vi "log analysis_gps.vi"() -> ()   [LabVIEW 2019] (continued)
INS_RTKFIXED,37.37077766145,126.72401317567,9.8633,22.3000,-0.2009,0.2209,0.0247,-0.192396038,1.572189477,119.250218807,0.6084,0.3900,0.7185,0.1389,0.1090,0.0824,0.1462,0.1512,5.0046,0f000001,0*0ea2a365\n\t", "INSPVAXA,USB3,0,52.5,FINESTEERING,2107,282225.550,02000000,471d,15824;INS_ALIGNMENT_COMPLETE,INS_RTKFIXED,37.37077734941,126.72401466448,9.8621,22.3000,-0.1997,0.2260,0.0207,-0.108448502,1.711031011,118.230862766,0.6084,0.3900,0.7185,0.1389,0.1090,0.0824,0.1462,0.1512,5.0046,0f000001,0*0e52b076\n\t", "INSPVAXA,USB3,0,48.5,FINESTEERING,2107,282226.050,02000000,471d,15824;INS_ALIGNMENT_COMPLETE,INS_RTKFIXED,37.37077704777,126.72401614595,9.8618,22.3000,-0.1720,0.2084,0.0247,-0.161231391,1.488834735,117.043709795,0.5373,0.3399,0.6690,0.1307,0.1036,0.0789,0.1454,0.1502,5.0054,0f000001,0*01dce4f3\n\t", "INSPVAXA,USB3,0,48.5,FINESTEERING,2107,282227.050,02000000,471d,15824;INS_ALIGNMENT_COMPLETE,INS_RTKFIXED,37.37077593278,126.72401891596,9.8631,22.3000,-0.1697,0.2262,0.0181,-0.178975170,1.493639019,115.812677176,0.5005,0.3171,0.6343,0.1279,0.1027,0.0771,0.1451,0.1499,5.0056,0f000001,0*b5f48b56\n\t", "INSPVAXA,USB3,0,51.0,FINESTEERING,2107,282227.550,02000000,471d,15824;INS_ALIGNMENT_COMPLETE,INS_RTKFIXED,37.37077534199,126.72402027291,9.8655,22.3000,-0.1792,0.2154,0.0259,-0.205196219,1.587681370,115.700553222,0.5005,0.3171,0.6343,0.1279,0.1027,0.0771,0.1451,0.1499,5.0056,0f000001,0*9a4eb5a2\n\t", "INSPVAXA,USB3,0,51.0,FINESTEERING,2107,282228.050,02000000,471d,15824;INS_ALIGNMENT_COMPLETE,INS_RTKFIXED,37.37077473925,126.72402159293,9.8669,22.3000,-0.1676,0.2065,0.0190,-0.168899804,1.509556154,115.821588566,0.4803,0.3065,0.6087,0.1271,0.1026,0.0763,0.1447,0.1496,5.0053,0f000001,0*25784804\n\t", "INSPVAXA,USB3,0,52.5,FINESTEERING,2107,282228.550,02000000,471d,15824;INS_ALIGNMENT_COMPLETE,INS_RTKFIXED,37.37077412906,126.72402288572,9.8668,22.3000,-0.1602,0.2130,0.0258,-0.196596636,1.388177172,115.979386072,0.4803,0.3065,0.6087,0.1271,0.1026,0.0763,0.1447,0.1496,5.0053,0f000001,0*cbeb8b2e\n\t", "INSPVAXA,USB3,0,50.5,FINESTEERING,2107,282229.050,02000000,471d,15824;INS_ALIGNMENT_COMPLETE,INS_RTKFIXED,37.37077350628,126.72402417744,9.8684,22.3000,-0.1816,0.2229,0.0203,-0.296207057,1.402486363,116.142608902,0.4697,0.3022,0.5898,0.1268,0.1020,0.0761,0.1442,0.1494,5.0046,0f000001,0*7993bda1\n\t", "INSPVAXA,USB3,0,50.5,FINESTEERING,2107,282229.550,02000000,471d,15824;INS_ALIGNMENT_COMPLETE,INS_RTKFIXED,37.37077278657,126.72402567791,9.8734,22.3000,-0.1941,0.2532,0.0237,-0.163503095,1.302197748,116.467398077,0.4697,0.3022,0.5898,0.1268,0.1020,0.0761,0.1442,0.1494,5.0046,0f000001,0*18de387b\n\t", "INSPVAXA,USB3,0,50.5,FINESTEERING,2107,282230.050,02000000,471d,15824;INS_ALIGNMENT_COMPLETE,INS_RTKFIXED,37.37077205146,126.72402713587,9.8769,22.3000,-0.1969,0.2300,0.0189,-0.143209861,1.267665510,116.875874478,0.4697,0.3022,0.5898,0.1268,0.1020,0.0761,0.1442,0.1494,5.0046,0f000001,0*6a8b4120\n\t", "INSPVAXA,USB3,0,50.5,FINESTEERING,2107,282231.050,02000000,471d,15824;INS_ALIGNMENT_COMPLETE,INS_RTKFIXED,37.37077037953,126.72402966350,9.8905,22.3000,-0.1831,0.2077,0.0203,-0.481877841,1.390379497,118.801399041,0.5188,0.3394,0.6182,0.1322,0.1054,0.0787,0.1443,0.1499,5.0038,0f000001,0*a6adcd9b\n\t", "INSPVAXA,USB3,0,51.0,FINESTEERING,2107,282231.550,02000000,471d,15824;INS_ALIGNMENT_COMPLETE,INS_RTKFIXED,37.37076971531,126.72403108088,9.8920,22.3000,-0.2013,0.2070,0.0109,-0.551553251,1.424964992,120.007848450,0.5188,0.3394,0.6182,0.1322,0.1054,0.0787,0.1443,0.1499,5.0038,0f000001,0*6cb6a544\n\t", "INSPVAXA,USB3,0,48.0,FINESTEERING,2107,282232.550,02000000,471d,15824;INS_ALIGNMENT_COMPLETE,INS_RTKFIXED,37.37076823474,126.72403383781,9.8941,22.3000,-0.2085,0.2221,0.0077,-0.388348000,1.567603173,122.220869009,0.4952,0.3205,0.5986,0.1271,0.0996,0.0779,0.1435,0.1490,5.0025,0f000001,0*80bf9f92\n\t", "INSPVAXA,USB3,0,50.0,FINESTEERING,2107,282233.550,02000000,471d,15824;INS_ALIGNMENT_COMPLETE,INS_RTKFIXED,37.37076641843,126.72403639264,9.9004,22.3000,-0.2178,0.2114,0.0096,-0.342808402,1.379099654,123.844356856,0.4952,0.3205,0.5986,0.1271,0.0996,0.0779,0.1435,0.1490,5.0025,0f000001,0*b00cd8f2\n\t", "INSPVAXA,USB3,0,50.0,FINESTEERING,2107,282234.050,02000000,471d,15824;INS_ALIGNMENT_COMPLETE,INS_RTKFIXED,37.37076539646,126.72403759594,9.9065,22.3000,-0.2225,0.2060,0.0095,-0.323054638,1.365837565,124.363784031,0.4952,0.3205,0.5986,0.1271,0.0996,0.0779,0.1435,0.1490,5.0025,0f000001,0*63b70899\n\t", "INSPVAXA,USB3,0,52.5,FINESTEERING,2107,282235.050,02000000,471d,15824;INS_ALIGNMENT_COMPLETE,INS_RTKFIXED,37.37076332295,126.72403997269,9.9185,22.3000,-0.2405,0.1895,0.0090,-0.183163482,1.364210608,124.971240350,0.5787,0.3754,0.6724,0.1350,0.1055,0.0817,0.1450,0.1501,5.0042,0f000001,0*0695c6fe\n\t", "INSPVAXA,USB3,0,52.5,FINESTEERING,2107,282235.550,02000000,471d,15824;INS_ALIGNMENT_COMPLETE,INS_RTKFIXED,37.37076275238,126.72404129303,9.9173,22.3000,-0.2324,0.1950,0.0071,-0.186698701,1.433095959,125.178228053,0.5787,0.3754,0.6724,0.1350,0.1055,0.0817,0.1450,0.1501,5.0042,0f000001,0*22a772a5\n\t", "INSPVAXA,USB3,0,51.0,FINESTEERING,2107,282236.050,02000000,471d,15824;INS_ALIGNMENT_COMPLETE,INS_RTKFIXED,37.37076213061,126.72404264687,9.9162,22.3000,-0.2356,0.2149,0.0160,-0.109376323,1.538913747,125.183228459,0.5240,0.3345,0.6382,0.1270,0.0999,0.0792,0.1443,0.1492,5.0048,0f000001,0*e39a076f\n\t", "INSPVAXA,USB3,0,51.0,FINESTEERING,2107,282237.050,02000000,471d,15824;INS_ALIGNMENT_COMPLETE,INS_RTKFIXED,37.37076053615,126.72404538521,9.9185,22.3000,-0.2398,0.2523,0.0058,-0.149955432,1.536125900,125.085519397,0.4941,0.3144,0.6129,0.1240,0.0987,0.0779,0.1441,0.1488,5.0061,0f000001,0*b0cbabaf\n\t", "INSPVAXA,USB3,0,49.0,FINESTEERING,2107,282238.050,02000000,471d,15824;INS_ALIGNMENT_COMPLETE,INS_RTKFIXED,37.37075892495,126.72404799622,9.9275,22.3000,-0.2194,0.2349,0.0204,-0.036624693,1.339643543,124.302497248,0.4765,0.3044,0.5938,0.1228,0.0987,0.0772,0.1439,0.1487,5.0076,0f000001,0*d84ea5b6\n\t", "INSPVAXA,USB3,0,49.0,FINESTEERING,2107,282239.050,02000000,471d,15824;INS_ALIGNMENT_COMPLETE,INS_RTKFIXED,37.37075731633,126.72405060135,9.9337,22.3000,-0.2234,0.2366,0.0085,-0.038602813,1.211050362,123.083406673,0.4672,0.3000,0.5797,0.1224,0.0986,0.0769,0.1436,0.1486,5.0092,0f000001,0*2a044e17\n\t", "INSPVAXA,USB3,0,52.5,FINESTEERING,2107,282240.050,02000000,471d,15824;INS_ALIGNMENT_COMPLETE,INS_RTKFIXED,37.37075580155,126.72405321567,9.9361,22.3000,-0.2036,0.2395,0.0145,-0.175150317,1.281192873,121.711657184,0.4620,0.2982,0.5691,0.1221,0.0979,0.0769,0.1433,0.1484,5.0109,0f000001,0*31735912\n\t", "INSPVAXA,USB3,0,52.0,FINESTEERING,2107,282240.550,02000000,471d,15824;INS_ALIGNMENT_COMPLETE,INS_RTKFIXED,37.37075505273,126.72405453213,9.9380,22.3000,-0.2095,0.2475,0.0059,-0.133753229,1.305172300,121.169613627,0.4620,0.2982,0.5691,0.1221,0.0979,0.0769,0.1433,0.1484,5.0109,0f000001,0*e864ebce\n\t", "INSPVAXA,USB3,0,48.5,FINESTEERING,2107,282243.050,02000000,471d,15824;INS_ALIGNMENT_COMPLETE,INS_RTKFIXED,37.37075099194,126.72406136178,9.9623,22.3000,-0.1962,0.2522,0.0127,-0.046095058,0.957232384,119.664456339,0.5142,0.3357,0.6005,0.1273,0.1006,0.0797,0.1435,0.1490,5.0157,0f000001,0*ddc696cd\n\t", "INSPVAXA,USB3,0,48.0,FINESTEERING,2107,282243.550,02000000,471d,15824;INS_ALIGNMENT_COMPLETE,INS_RTKFIXED,37.37075036511,126.72406264733,9.9641,22.3000,-0.1945,0.2497,0.0107,-0.063490953,0.947400713,119.636674206,0.5142,0.3357,0.6005,0.1273,0.1006,0.0797,0.1435,0.1490,5.0157,0f000001,0*2c22af95\n\t", "INSPVAXA,USB3,0,50.0,FINESTEERING,2107,282246.550,02000000,471d,15824;INS_ALIGNMENT_COMPLETE,INS_RTKFIXED,37.37074619554,126.72407050516,9.9901,22.3000,-0.1782,0.2479,0.0044,0.220698175,1.278945577,119.830464589,0.4789,0.3066,0.5774,0.1203,0.0946,0.0781,0.1428,0.1481,5.0182,0f000001,0*b4ea3089\n\t", "INSPVAXA,USB3,0,51.0,FINESTEERING,2107,282261.600,02008000,471d,15824;INS_ALIGNMENT_COMPLETE,INS_RTKFIXED,37.37072301964,126.72410864198,10.0789,22.3000,-0.1970,0.2354,0.0160,-0.160873741,1.322866529,121.119514583,0.4897,0.3148,0.6247,0.1298,0.1039,0.0767,0.1436,0.1490,5.0292,0f000001,0*85434b09\n\t", "INSPVAXA,USB3,0,50.5,FINESTEERING,2107,282262.100,02008000,471d,15824;INS_ALIGNMENT_COMPLETE,INS_RTKFIXED,37.37072222272,126.72410992724,10.0823,22.3000,-0.1883,0.2369,0.0121,0.011480682,1.244674277,120.532236713,0.5693,0.3742,0.6825,0.1391,0.1098,0.0808,0.1445,0.1502,5.0254,0f000001,0*eae9fcde\n\t", "INSPVAXA,USB3,0,49.5,FINESTEERING,2107,282266.600,02000000,471d,15824;INS_ALIGNMENT_COMPLETE,INS_RTKFIXED,37.37071564001,126.72412194317,10.1142,22.3000,-0.1803,0.2485,0.0162,-0.167874326,0.987777383,118.589325472,0.4588,0.3004,0.5750,0.1240,0.0989,0.0769,0.1427,0.1481,5.0170,0f000001,0*94bf16e1\n\t", "INSPVAXA,USB3,0,51.5,FINESTEERING,2107,282267.100,02000000,471d,15824;INS_ALIGNMENT_COMPLETE,INS_RTKFIXED,37.37071488193,126.72412330620,10.1185,22.3000,-0.1782,0.2546,0.0105,-0.234897053,0.733993944,118.660329802,0.4588,0.3004,0.5750,0.1240,0.0989,0.0769,0.1427,0.1481,5.0170,0f000001,0*405246e9\n\t", "INSPVAXA,USB3,0,50.5,FINESTEERING,2107,282268.100,02000000,471d,15824;INS_ALIGNMENT_COMPLETE,INS_RTKFIXED,37.37071326261,126.72412602696,10.1265,22.3000,-0.1797,0.2316,0.0106,-0.308837193,0.760008710,118.874107108,0.4588,0.3004,0.5750,0.1240,0.0989,0.0769,0.1427,0.1481,5.0170,0f000001,0*38424b3d\n\t", "INSPVAXA,USB3,0,50.5,FINESTEERING,2107,282268.600,02000000,471d,15824;INS_ALIGNMENT_COMPLETE,INS_RTKFIXED,37.37071245816,126.72412735967,10.1316,22.3000,-0.1815,0.2421,0.0127,-0.377106953,0.735852772,118.906106803,0.4588,0.3004,0.5750,0.1240,0.0989,0.0769,0.1427,0.1481,5.0170,0f000001,0*11ddd4c2\n\t", "INSPVAXA,USB3,0,50.0,FINESTEERING,2107,282269.600,02000000,471d,15824;INS_ALIGNMENT_COMPLETE,INS_RTKFIXED,37.37071107493,126.72412999444,10.1387,22.3000,-0.1723,0.2314,0.0190,-0.521024846,1.079546483,119.280736819,0.5511,0.3672,0.6510,0.1337,0.1063,0.0814,0.1442,0.1496,5.0179,0f000001,0*5d398b6e\n\t", "INSPVAXA,USB3,0,51.0,FINESTEERING,2107,282270.600,02008000,471d,15824;INS_ALIGNMENT_COMPLETE,INS_RTKFIXED,37.37070978971,126.72413254865,10.1460,22.3000,-0.1852,0.2381,0.0080,-0.437420088,1.249078779,119.796376349,0.5043,0.3305,0.6212,0.1261,0.1003,0.0792,0.1434,0.1486,5.0184,0f000001,0*9b5f8ba6\n\t", "INSPVAXA,USB3,0,47.5,FINESTEERING,2107,282271.100,02008000,471d,15824;INS_ALIGNMENT_COMPLETE,INS_RTKFIXED,37.37070909074,126.72413388392,10.1504,22.3000,-0.1800,0.2456,0.0054,-0.539837627,1.179431865,120.094630407,0.4787,0.3123,0.5991,0.1229,0.0985,0.0779,0.1432,0.1482,5.0193,0f000001,0*40acc907\n\t", "INSPVAXA,USB3,0,47.5,FINESTEERING,2107,282271.600,02008000,471d,15824;INS_ALIGNMENT_COMPLETE,INS_RTKFIXED,37.37070834780,126.72413522387,10.1531,22.3000,-0.1652,0.2443,0.0195,-0.572032410,1.056169102,120.353350938,0.4787,0.3123,0.5991,0.1229,0.0985,0.0779,0.1432,0.1482,5.0193,0f000001,0*1c071485\n\t", "INSPVAXA,USB3,0,48.5,FINESTEERING,2107,282272.600,02008000,471d,15824;INS_ALIGNMENT_COMPLETE,INS_RTKFIXED,37.37070676202,126.72413789177,10.1597,22.3000,-0.1767,0.2382,0.0118,-0.374820510,0.656096150,120.799348362,0.4787,0.3123,0.5991,0.1229,0.0985,0.0779,0.1432,0.1482,5.0193,0f000001,0*9be2d9dc\n\t", "INSPVAXA,USB3,0,51.5,FINESTEERING,2107,282273.600,02008000,471d,15824;INS_ALIGNMENT_COMPLETE,INS_RTKFIXED,37.37070511778,126.72414055042,10.1715,22.3000,-0.1870,0.2363,0.0134,-0.459769985,0.798437213,121.336357877,0.4787,0.3123,0.5991,0.1229,0.0985,0.0779,0.1432,0.1482,5.0193,0f000001,0*703348aa\n\t", "INSPVAXA,USB3,0,50.0,FINESTEERING,2107,282274.600,02000000,471d,15824;INS_ALIGNMENT_COMPLETE,INS_RTKFIXED,37.37070363879,126.72414308570,10.1749,22.3000,-0.1813,0.2312,0.0078,-0.604469553,1.084486216,121.923542581,0.5575,0.3692,0.6704,0.1333,0.1077,0.0814,0.1446,0.1496,5.0225,0f000001,0*5c099128\n\t", "INSPVAXA,USB3,0,50.5,FINESTEERING,2107,282275.100,02000000,471d,15824;INS_ALIGNMENT_COMPLETE,INS_RTKFIXED,37.37070296140,126.72414429321,10.1745,22.3000,-0.1748,0.2312,0.0107,-0.634765121,1.047187447,122.187120855,0.5046,0.3310,0.6337,0.1261,0.1021,0.0787,0.1438,0.1486,5.0224,0f000001,0*d0387721\n\t", "INSPVAXA,USB3,0,50.5,FINESTEERING,2107,282275.600,02000000,471d,15824;INS_ALIGNMENT_COMPLETE,INS_RTKFIXED,37.37070222382,126.72414554188,10.1759,22.3000,-0.1770,0.2216,0.0167,-0.613341338,0.949181726,122.390549431,0.5046,0.3310,0.6337,0.1261,0.1021,0.0787,0.1438,0.1486,5.0224,0f000001,0*c2bde323\n\t", "INSPVAXA,USB3,0,49.0,FINESTEERING,2107,282276.100,02000000,471d,15824;INS_ALIGNMENT_COMPLETE,INS_RTKFIXED,37.37070146570,126.72414680907,10.1773,22.3000,-0.1774,0.2243,0.0157,-0.609174519,0.899706635,122.569585175,0.4767,0.3125,0.6072,0.1235,0.1004,0.0773,0.1434,0.1482,5.0223,0f000001,0*a35fb81b\n\t", "INSPVAXA,USB3,0,50.0,FINESTEERING,2107,282277.100,02000000,471d,15824;INS_ALIGNMENT_COMPLETE,INS_RTKFIXED,37.37069991504,126.72414929974,10.1840,22.3000,-0.1767,0.2226,0.0047,-0.557997930,0.665249909,123.001928540,0.4767,0.3125,0.6072,0.1235,0.1004,0.0773,0.1434,0.1482,5.0223,0f000001,0*cb3103e7\n\t", "INSPVAXA,USB3,0,53.0,FINESTEERING,2107,282278.100,02000000,471d,15824;INS_ALIGNMENT_COMPLETE,INS_RTKFIXED,37.37069823681,126.72415183772,10.1961,22.3000,-0.1823,0.2204,0.0074,-0.523658025,0.566082067,123.287197308,0.4767,0.3125,0.6072,0.1235,0.1004,0.0773,0.1434,0.1482,5.0223,0f000001,0*25d51a4b\n\t", "INSPVAXA,USB3,0,47.5,FINESTEERING,2107,282280.100,02000000,471d,15824;INS_ALIGNMENT_COMPLETE,INS_RTKFIXED,37.37069498335,126.72415703248,10.2090,22.3000,-0.1979,0.2492,0.0153,-0.691574925,0.436072461,123.457665548,0.5547,0.3701,0.6738,0.1343,0.1087,0.0808,0.1445,0.1496,5.0239,0f000001,0*1cc0a1a6\n\t", "INSPVAXA,USB3,0,49.5,FINESTEERING,2107,282281.100,02000000,471d,15824;INS_ALIGNMENT_COMPLETE,INS_RTKFIXED,37.37069324003,126.72415967576,10.2193,22.3000,-0.1883,0.2410,0.0110,-0.444587067,-0.239892052,123.232720595,0.5547,0.3701,0.6738,0.1343,0.1087,0.0808,0.1445,0.1496,5.0239,0f000001,0*fc1f5c5f\n\t", "INSPVAXA,USB3,0,47.5,FINESTEERING,2107,282282.100,02000000,471d,15824;INS_ALIGNMENT_COMPLETE,INS_RTKFIXED,37.37069160850,126.72416229361,10.2264,22.3000,-0.1858,0.2281,-0.0001,-0.736056303,-0.906540815,122.497361054,0.5875,0.3887,0.7203,0.1380,0.1105,0.0818,0.1447,0.1498,5.0279,0f000001,0*0c5128b7\n\t", "INSPVAXA,USB3,0,47.5,FINESTEERING,2107,282282.600,02000000,471d,15824;INS_ALIGNMENT_COMPLETE,INS_RTKFIXED,37.37069089697,126.72416351730,10.2196,22.3000,-0.1871,0.2326,0.0042,-0.425257190,-0.862348838,121.960644857,0.5875,0.3887,0.7203,0.1380,0.1105,0.0818,0.1447,0.1498,5.0279,0f000001,0*490a0fa5\n\t", "INSPVAXA,USB3,0,46.5,FINESTEERING,2107,282283.600,02008000,471d,15824;INS_ALIGNMENT_COMPLETE,INS_RTKFIXED,37.37068940958,126.72416607579,10.2138,22.3000,-0.1636,0.2189,-0.0003,-0.120036604,-0.860841459,120.892387916,0.5875,0.3887,0.7203,0.1380,0.1105,0.0818,0.1447,0.1498,5.0279,0f000001,0*9192f1a2\n\t", "INSPVAXA,USB3,0,51.5,FINESTEERING,2107,282284.100,02008000,471d,15824;INS_ALIGNMENT_COMPLETE,INS_RTKFIXED,37.37068864878,126.72416738015,10.2177,22.3000,-0.1641,0.2313,0.0038,-0.033754752,-0.589658100,120.436095799,0.5875,0.3887,0.7203,0.1380,0.1105,0.0818,0.1447,0.1498,5.0279,0f000001,0*0148cd2e\n\t", "INSPVAXA,USB3,0,51.5,FINESTEERING,2107,282284.600,02008000,471d,15824;INS_ALIGNMENT_COMPLETE,INS_RTKFIXED,37.37068791248,126.72416871170,10.2207,22.3000,-0.1613,0.2366,0.0105,-0.227472838,-0.490349868,119.960742273,0.5875,0.3887,0.7203,0.1380,0.1105,0.0818,0.1447,0.1498,5.0279,0f000001,0*af559696\n\t", "INSPVAXA,USB3,0,51.5,FINESTEERING,2107,282285.100,02008000,471d,15824;INS_ALIGNMENT_COMPLETE,INS_RTKFIXED,37.37068720846,126.72417000092,10.2252,22.3000,-0.1602,0.2440,0.0066,-0.187971792,0.385088793,119.635511852,0.5949,0.3921,0.7470,0.1392,0.1132,0.0817,0.1449,0.1501,5.0298,0f000001,0*026b0f4f\n\t", "INSPVAXA,USB3,0,52.0,FINESTEERING,2107,282285.600,02008000,471d,15824;INS_ALIGNMENT_COMPLETE,INS_RTKFIXED,37.37068652184,126.72417128801,10.2137,22.3000,-0.1658,0.2472,-0.0117,-0.055492896,0.657869792,119.429156162,0.5949,0.3921,0.7470,0.1392,0.1132,0.0817,0.1449,0.1501,5.0298,0f000001,0*cfd09dcb\n\t", "INSPVAXA,USB3,0,48.5,FINESTEERING,2107,282286.100,02008000,471d,15824;INS_ALIGNMENT_COMPLETE,INS_RTKFIXED,37.37068585553,126.72417255759,10.2052,22.3000,-0.1551,0.2284,0.0107,-0.089152312,0.639970928,119.250576511,0.5190,0.3392,0.6809,0.1320,0.1082,0.0780,0.1441,0.1491,5.0307,0f000001,0*ec53885d\n\t", "INSPVAXA,USB3,0,48.5,FINESTEERING,2107,282286.600,02008000,471d,15824;INS_ALIGNMENT_COMPLETE,INS_RTKFIXED,37.37068514150,126.72417389818,10.2001,22.3000,-0.1412,0.2197,0.0066,0.024364093,0.832001131,119.298455875,0.5190,0.3392,0.6809,0.1320,0.1082,0.0780,0.1441,0.1491,5.0307,0f000001,0*de9bf723\n\t", "INSPVAXA,USB3,0,48.5,FINESTEERING,2107,282287.100,02008000,471d,15824;INS_ALIGNMENT_COMPLETE,INS_RTKFIXED,37.37068448744,126.72417519191,10.1977,22.3000,-0.1331,0.1859,0.0151,-0.327488179,0.840633219,119.294501197,0.4827,0.3161,0.6365,0.1297,0.1073,0.0763,0.1436,0.1487,5.0297,0f000001,0*ec0356ba\n\t", "INSPVAXA,USB3,0,49.5,FINESTEERING,2107,282287.600,02000000,471d,15824;INS_ALIGNMENT_COMPLETE,INS_RTKFIXED,37.37068376486,126.72417656780,10.2009,22.3000,-0.1622,0.2304,0.0144,-0.264314636,1.151154189,119.357397918,0.4827,0.3161,0.6365,0.1297,0.1073,0.0763,0.1436,0.1487,5.0297,0f000001,0*1ac61951\n\t", "INSPVAXA,USB3,0,52.0,FINESTEERING,2107,282288.100,02000000,471d,15824;INS_ALIGNMENT_COMPLETE,INS_RTKFIXED,37.37068313188,126.72417778864,10.2013,22.3000,-0.1464,0.2451,0.0101,-0.437974736,2.271326824,119.414001695,0.4827,0.3161,0.6365,0.1297,0.1073,0.0763,0.1436,0.1487,5.0297,0f000001,0*f8a30918\n\t", "INSPVAXA,USB3,0,52.0,FINESTEERING,2107,282288.600,02000000,471d,15824;INS_ALIGNMENT_COMPLETE,INS_RTKFIXED,37.37068248207,126.72417903271,10.2071,22.3000,-0.1554,0.2479,0.0102,-0.520482478,3.090095843,119.464562963,0.4827,0.3161,0.6365,0.1297,0.1073,0.0763,0.1436,0.1487,5.0297,0f000001,0*4436d63b\n\t", "INSPVAXA,USB3,0,48.0,FINESTEERING,2107,282289.100,02000000,471d,15824;INS_ALIGNMENT_COMPLETE,INS_RTKFIXED,37.37068179402,126.72418031784,10.2124,22.3000,-0.1466,0.2345,0.0076,-0.435594765,3.881928783,119.627439178,0.5155,0.3438,0.6451,0.1390,0.1110,0.0782,0.1436,0.1489,5.0203,0f000001,0*d705b298\n\t", "INSPVAXA,USB3,0,48.0,FINESTEERING,2107,282289.600,02000000,471d,15824;INS_ALIGNMENT_COMPLETE,INS_RTKFIXED,37.37068106233,126.72418156036,10.2167,22.3000,-0.1573,0.2453,0.0197,-0.196955820,4.346907241,119.830177459,0.5155,0.3438,0.6451,0.1390,0.1110,0.0782,0.1436,0.1489,5.0203,0f000001,0*c638875e\n\t", "INSPVAXA,USB3,0,45.0,FINESTEERING,2107,282290.100,02000000,471d,15824;INS_ALIGNMENT_COMPLETE,INS_RTKFIXED,37.37068031183,126.72418287504,10.2233,22.3000,-0.1663,0.2481,0.0180,-0.098835981,4.376797831,120.158403122,0.5155,0.3438,0.6451,0.1390,0.1110,0.0782,0.1436,0.1489,5.0203,0f000001,0*f931a41f\n\t", "INSPVAXA,USB3,0,45.0,FINESTEERING,2107,282290.600,02000000,471d,15824;INS_ALIGNMENT_COMPLETE,INS_RTKFIXED,37.37067956238,126.72418428483,10.2337,22.3000,-0.1707,0.2482,0.0265,-0.202932482,4.159469739,120.506147685,0.5155,0.3438,0.6451,0.1390,0.1110,0.0782,0.1436,0.1489,5.0203,0f000001,0*908c714d\n\t", "INSPVAXA,USB3,0,45.0,FINESTEERING,2107,282291.100,02000000,471d,15824;INS_ALIGNMENT_COMPLETE,INS_RTKFIXED,37.37067879937,126.72418567734,10.2444,22.3000,-0.1651,0.2543,0.0207,-0.251060851,3.844476935,120.878401990,0.5409,0.3575,0.6537,0.1355,0.1073,0.0795,0.1434,0.1485,4.9849,0f000001,0*d6642fae\n\t", "INSPVAXA,USB3,0,49.0,FINESTEERING,2107,282291.600,02000000,471d,15824;INS_ALIGNMENT_COMPLETE,INS_RTKFIXED,37.37067799408,126.72418700521,10.2537,22.3000,-0.1763,0.2581,0.0156,-0.182414041,3.404030284,121.216304080,0.5409,0.3575,0.6537,0.1355,0.1073,0.0795,0.1434,0.1485,4.9849,0f000001,0*0bbc7934\n\t", "INSPVAXA,USB3,0,45.5,FINESTEERING,2107,282292.100,02000000,471d,15824;INS_ALIGNMENT_COMPLETE,INS_RTKFIXED,37.37067717574,126.72418831770,10.2613,22.3000,-0.1798,0.2515,0.0164,-0.016177386,3.020104731,121.543147805,0.5007,0.3269,0.6199,0.1278,0.1011,0.0781,0.1427,0.1475,4.9679,0f000001,0*266eeccf\n\t", "INSPVAXA,USB3,0,45.5,FINESTEERING,2107,282292.600,02000000,471d,15824;INS_ALIGNMENT_COMPLETE,INS_RTKFIXED,37.37067636900,126.72418961762,10.2690,22.3000,-0.1769,0.2534,0.0080,-0.042843128,2.826759878,121.907768191,0.5007,0.3269,0.6199,0.1278,0.1011,0.0781,0.1427,0.1475,4.9679,0f000001,0*aaae4f23\n\t", "INSPVAXA,USB3,0,45.5,FINESTEERING,2107,282293.100,02000000,471d,15824;INS_ALIGNMENT_COMPLETE,INS_RTKFIXED,37.37067553892,126.72419093232,10.2760,22.3000,-0.1811,0.2495,0.0116,-0.008430473,2.413814082,122.277222921,0.4766,0.3108,0.5954,0.1241,0.0990,0.0774,0.1425,0.1470,4.9617,0f000001,0*c888aeda\n\t", "INSPVAXA,USB3,0,46.5,FINESTEERING,2107,282293.600,02000000,471d,15824;INS_ALIGNMENT_COMPLETE,INS_RTKFIXED,37.37067472793,126.72419224415,10.2820,22.3000,-0.1803,0.2324,0.0113,-0.180884788,2.125088791,122.585479065,0.4766,0.3108,0.5954,0.1241,0.0990,0.0774,0.1425,0.1470,4.9617,0f000001,0*8a54f30e\n\t", "INSPVAXA,USB3,0,46.5,FINESTEERING,2107,282294.100,02008000,471d,15824;INS_ALIGNMENT_COMPLETE,INS_RTKFIXED,37.37067392240,126.72419354245,10.2863,22.3000,-0.1909,0.2309,0.0096,-0.404437997,1.924119291,122.825127987,0.4614,0.3022,0.5776,0.1224,0.0977,0.0772,0.1423,0.1468,4.9609,0f000001,0*f2faedc4\n\t", "DUALANTENNAHEADINGA,USB3,0,47.0,FINESTEERING,2107,282294.600,02008000,d426,15824;SOL_COMPUTED,NARROW_FLOAT,-1.000000000,121.189437866,-60.258087158,0.0,360.000000000,180.000000000,\"631T\",18,7,7,5,04,00,20,03*d581effc\n\t", "DUALANTENNAHEADINGA,USB3,0,45.0,FINESTEERING,2107,282295.100,02008000,d426,15824;SOL_COMPUTED,L1_FLOAT,-1.000000000,102.362266541,-42.452087402,0.0,360.000000000,180.000000000,\"631T\",17,6,6,3,04,00,20,01*c6a3d1e1\n\t", "DUALANTENNAHEADINGA,USB3,0,45.0,FINESTEERING,2107,282295.600,02008000,d426,15824;SOL_COMPUTED,L1_FLOAT,-1.000000000,103.041458130,-42.702667236,0.0,360.000000000,180.000000000,\"631T\",15,6,6,3,04,00,20,01*07943439\n\t", "INSPVAXA,USB3,0,45.5,FINESTEERING,2107,282296.100,02008000,471d,15824;INS_ALIGNMENT_COMPLETE,INS_RTKFIXED,37.37067068708,126.72419852812,10.3007,22.3000,-0.1831,0.2265,0.0055,-1.180023346,1.380731558,123.921580343,0.4463,0.2958,0.5559,0.1206,0.0957,0.0774,0.1421,0.1465,4.9614,0f000001,0*6538f2e2\n\t", "DUALANTENNAHEADINGA,USB3,0,45.5,FINESTEERING,2107,282296.600,02008000,d426,15824;INSUFFICIENT_OBS,NONE,0.000000000,0.000000000,0.000000000,0.0,0.000000000,0.000000000,\"\",0,0,0,0,00,00,00,00*630506ca\n\t", "INSPVAXA,USB3,0,50.5,FINESTEERING,2107,282297.100,02008000,471d,15824;INS_ALIGNMENT_COMPLETE,INS_RTKFIXED,37.37066909241,126.72420090990,10.3083,22.3000,-0.1861,0.2064,0.0054,-1.451232970,2.139492751,124.282872789,0.4463,0.2958,0.5559,0.1206,0.0957,0.0774,0.1421,0.1465,4.9614,0f000001,0*92259f00\n\t", "INSPVAXA,USB3,0,50.5,FINESTEERING,2107,282297.600,02008000,471d,15824;INS_ALIGNMENT_COMPLETE,INS_RTKFIXED,37.37066824319,126.72420217982,10.3132,22.3000,-0.1844,0.2206,0.0132,-1.291295595,2.299474120,124.306238371,0.4463,0.2958,0.5559,0.1206,0.0957,0.0774,0.1421,0.1465,4.9614,0f000001,0*08710687\n\t", "INSPVAXA,USB3,0,47.5,FINESTEERING,2107,282298.100,02000000,471d,15824;INS_ALIGNMENT_COMPLETE,INS_RTKFIXED,37.37066736588,126.72420348765,10.3177,22.3000,-0.2044,0.2368,0.0054,-0.934530380,2.484268060,124.268578123,0.4463,0.2958,0.5559,0.1206,0.0957,0.0774,0.1421,0.1465,4.9614,0f000001,0*e22edcc5\n\t", "INSPVAXA,USB3,0,47.5,FINESTEERING,2107,282298.600,02000000,471d,15824;INS_ALIGNMENT_COMPLETE,INS_RTKFIXED,37.37066650414,126.72420478717,10.3223,22.3000,-0.2012,0.2369,0.0184,-0.644074301,2.480545222,124.200345870,0.4463,0.2958,0.5559,0.1206,0.0957,0.0774,0.1421,0.1465,4.9614,0f000001,0*352785c6\n\t", "DUALANTENNAHEADINGA,USB3,0,47.5,FINESTEERING,2107,282299.100,02000000,d426,15824;SOL_COMPUTED,L1_FLOAT,-1.000000000,104.413963318,-39.969207764,0.0,360.000000000,180.000000000,\"631T\",13,6,6,3,04,00,20,01*0865e994\n\t", "INSPVAXA,USB3,0,50.5,FINESTEERING,2107,282299.600,02000000,471d,15824;INS_ALIGNMENT_COMPLETE,INS_RTKFIXED,37.37066485429,126.72420728055,10.3338,22.3000,-0.1766,0.2255,0.0106,-0.427425360,2.613001308,123.918175159,0.5467,0.3647,0.6429,0.1311,0.1043,0.0822,0.1440,0.1485,4.9572,0f000001,0*9195cd30\n\t", "DUALANTENNAHEADINGA,USB3,0,48.5,FINESTEERING,2107,282300.100,02000000,d426,15824;INSUFFICIENT_OBS,NONE,0.000000000,0.000000000,0.000000000,0.0,0.000000000,0.000000000,\"\",0,0,0,0,00,00,00,00*e37ee9dd\n\t", "INSPVAXA,USB3,0,48.5,FINESTEERING,2107,282300.600,02000000,471d,15824;INS_ALIGNMENT_COMPLETE,INS_RTKFIXED,37.37066328709,126.72420961412,10.3498,22.3000,-0.1736,0.2244,0.0088,0.359177910,2.809986470,122.746384248,0.5045,0.3294,0.6194,0.1239,0.0993,0.0801,0.1433,0.1477,4.9538,0f000001,0*bd968cc8\n\t", "INSPVAXA,USB3,0,49.0,FINESTEERING,2107,282301.100,02000000,471d,15824;INS_ALIGNMENT_COMPLETE,INS_RTKFIXED,37.37066253151,126.72421082792,10.3582,22.3000,-0.1761,0.2216,0.0197,0.484810078,3.068722182,122.157081229,0.5045,0.3294,0.6194,0.1239,0.0993,0.0801,0.1433,0.1477,4.9538,0f000001,0*fc57e6fe\n\t", "DUALANTENNAHEADINGA,USB3,0,49.0,FINESTEERING,2107,282301.600,02000000,d426,15824;INSUFFICIENT_OBS,NONE,0.000000000,0.000000000,0.000000000,0.0,0.000000000,0.000000000,\"\",0,0,0,0,00,00,00,00*fb3df011\n\t", "DUALANTENNAHEADINGA,USB3,0,49.0,FINESTEERING,2107,282302.100,02000000,d426,15824;SOL_COMPUTED,NARROW_FLOAT,-1.000000000,117.785400391,-42.761993408,0.0,360.000000000,180.000000000,\"631T\",16,6,6,5,04,00,20,03*f6212de6\n\t", "INSPVAXA,USB3,0,51.5,FINESTEERING,2107,282302.600,02000000,471d,15824;INS_ALIGNMENT_COMPLETE,INS_RTKFIXED,37.37066035921,126.72421474502,10.3743,22.3000,-0.1596,0.2340,0.0126,0.411007245,2.764808403,120.160386775,0.5045,0.3294,0.6194,0.1239,0.0993,0.0801,0.1433,0.1477,4.9538,0f000001,0*7b8f0c3b\n\t", "DUALANTENNAHEADINGA,USB3,0,49.5,FINESTEERING,2107,282303.100,02000000,d426,15824;INSUFFICIENT_OBS,NONE,0.000000000,0.000000000,0.000000000,0.0,0.000000000,0.000000000,\"\",0,0,0,0,00,00,00,00*96d140e5\n\t", "DUALANTENNAHEADINGA,USB3,0,49.5,FINESTEERING,2107,282303.600,02000000,d426,15824;INSUFFICIENT_OBS,NONE,0.000000000,0.000000000,0.000000000,0.0,0.000000000,0.000000000,\"\",0,0,0,0,00,00,00,00*3f9a20d4\n\t", "INSPVAXA,USB3,0,43.0,FINESTEERING,2107,282304.100,02000000,471d,15824;INS_ALIGNMENT_COMPLETE,INS_RTKFIXED,37.37065823022,126.72421863146,10.4032,22.3000,-0.1537,0.2368,0.0051,0.137147576,2.044689982,118.905091584,0.5709,0.3745,0.6911,0.1341,0.1081,0.0826,0.1447,0.1492,4.9492,0f000001,0*2d96de96\n\t", "DUALANTENNAHEADINGA,USB3,0,43.0,FINESTEERING,2107,282304.600,02000000,d426,15824;INSUFFICIENT_OBS,NONE,0.000000000,0.000000000,0.000000000,0.0,0.000000000,0.000000000,\"\",0,0,0,0,00,00,00,00*c23e1cc5\n\t", "DUALANTENNAHEADINGA,USB3,0,43.0,FINESTEERING,2107,282305.100,02000000,d426,15824;SOL_COMPUTED,L1_FLOAT,-1.000000000,149.112899780,-55.880187988,0.0,360.000000000,180.000000000,\"631T\",16,6,6,5,04,00,20,03*c998c635\n\t", "INSPVAXA,USB3,0,50.0,FINESTEERING,2107,282305.600,02000000,471d,15824;INS_ALIGNMENT_COMPLETE,INS_RTKFIXED,37.37065621091,126.72422257875,10.4180,22.3000,-0.1470,0.2285,0.0045,0.107072470,2.040461539,118.820220655,0.5709,0.3745,0.6911,0.1341,0.1081,0.0826,0.1447,0.1492,4.9492,0f000001,0*28a83c0b\n\t", "DUALANTENNAHEADINGA,USB3,0,49.0,FINESTEERING,2107,282306.100,02000000,d426,15824;SOL_COMPUTED,NARROW_FLOAT,-1.000000000,131.179367065,-49.751617432,0.0,360.000000000,180.000000000,\"631T\",16,6,6,5,04,00,20,03*d544857e\n\t", "INSPVAXA,USB3,0,49.0,FINESTEERING,2107,282306.600,02000000,471d,15824;INS_ALIGNMENT_COMPLETE,INS_RTKFIXED,37.37065472577,126.72422510434,10.4346,22.3000,-0.1517,0.2382,0.0100,-0.069215248,2.129232392,118.969367736,0.5936,0.3892,0.7368,0.1380,0.1115,0.0828,0.1450,0.1498,4.9367,0f000001,0*a2c53eca\n\t", "DUALANTENNAHEADINGA,USB3,0,48.0,FINESTEERING,2107,282307.100,02000000,d426,15824;INSUFFICIENT_OBS,NONE,0.000000000,0.000000000,0.000000000,0.0,0.000000000,0.000000000,\"\",0,0,0,0,00,00,00,00*83621ed4\n\t", "DUALANTENNAHEADINGA,USB3,0,48.0,FINESTEERING,2107,282307.600,02000000,d426,15824;INSUFFICIENT_OBS,NONE,0.000000000,0.000000000,0.000000000,0.0,0.000000000,0.000000000,\"\",0,0,0,0,00,00,00,00*2a297ee5\n\t", "DUALANTENNAHEADINGA,USB3,0,48.0,FINESTEERING,2107,282308.100,02000000,d426,15824;SOL_COMPUTED,NARROW_FLOAT,-1.000000000,130.346817017,-46.744110107,0.0,360.000000000,180.000000000,\"631T\",13,6,6,5,04,00,20,03*2381209c\n\t", "DUALANTENNAHEADINGA,USB3,0,50.0,FINESTEERING,2107,282308.600,02000000,d426,15824;SOL_COMPUTED,NARROW_FLOAT,-1.000000000,131.524536133,-48.144073486,0.0,360.000000000,180.000000000,\"631T\",17,6,6,5,04,00,20,03*26d8279d\n\t", "INSPVAXA,USB3,0,50.0,FINESTEERING,2107,282309.100,02000000,471d,15824;INS_ALIGNMENT_COMPLETE,INS_RTKFIXED,37.37065087449,126.72423169405,10.4716,22.3000,-0.1818,0.2462,0.0157,-0.101661617,1.756669202,119.993193465,0.5316,0.3505,0.6792,0.1345,0.1096,0.0793,0.1439,0.1491,4.9301,0f000001,0*2fa2c19e\n\t", "INSPVAXA,USB3,0,50.5,FINESTEERING,2107,282309.600,02000000,471d,15824;INS_ALIGNMENT_COMPLETE,INS_RTKFIXED,37.37065005438,126.72423301384,10.4771,22.3000,-0.1715,0.2318,0.0129,-0.072761707,1.702932866,120.296688789,0.5316,0.3505,0.6792,0.1345,0.1096,0.0793,0.1439,0.1491,4.9301,0f000001,0*35eea818\n\t", "DUALANTENNAHEADINGA,USB3,0,50.0,FINESTEERING,2107,282310.100,02000000,d426,15824;INSUFFICIENT_OBS,NONE,0.000000000,0.000000000,0.000000000,0.0,0.000000000,0.000000000,\"\",0,0,0,0,00,00,00,00*14cc2e90\n\t", "INSPVAXA,USB3,0,50.0,FINESTEERING,2107,282310.600,02000000,471d,15824;INS_ALIGNMENT_COMPLETE,INS_RTKFIXED,37.37064838288,126.72423565428,10.4879,22.3000,-0.1825,0.2221,0.0118,0.275691228,1.663027619,120.773343582,0.5316,0.3505,0.6792,0.1345,0.1096,0.0793,0.1439,0.1491,4.9301,0f000001,0*997564fa\n\t", "DUALANTENNAHEADINGA,USB3,0,46.0,FINESTEERING,2107,282311.100,02000000,d426,15824;SOL_COMPUTED,NARROW_FLOAT,-1.000000000,117.813430786,-36.691406250,0.0,360.000000000,180.000000000,\"631T\",17,7,7,6,04,00,20,03*31d6dfd5\n\t", "DUALANTENNAHEADINGA,USB3,0,46.0,FINESTEERING,2107,282311.600,02000000,d426,15824;SOL_COMPUTED,NARROW_FLOAT,-1.000000000,120.262771606,-39.374176025,0.0,360.000000000,180.000000000,\"631T\",18,7,7,5,04,00,20,03*970c933d\n\t", "INSPVAXA,USB3,0,48.5,FINESTEERING,2107,282312.100,02000000,471d,15824;INS_ALIGNMENT_COMPLETE,INS_RTKFIXED,37.37064587490,126.72423949786,10.5026,22.3000,-0.1922,0.2292,0.0073,0.477048241,1.745843480,121.477542384,0.5806,0.3850,0.7206,0.1397,0.1125,0.0814,0.1439,0.1495,4.9286,0f000001,0*cdf8ddfc\n\t", "DUALANTENNAHEADINGA,USB3,0,48.5,FINESTEERING,2107,282312.600,02000000,d426,15824;INSUFFICIENT_OBS,NONE,0.000000000,0.000000000,0.000000000,0.0,0.000000000,0.000000000,\"\",0,0,0,0,00,00,00,00*914fc627\n\t", "INSPVAXA,USB3,0,48.0,FINESTEERING,2107,282313.100,02000000,471d,15824;INS_ALIGNMENT_COMPLETE,INS_RTKFIXED,37.37064429153,126.72424202455,10.5097,22.3000,-0.1991,0.2355,-0.0061,0.301334832,1.691394524,121.905200566,0.5806,0.3850,0.7206,0.1397,0.1125,0.0814,0.1439,0.1495,4.9286,0f000001,0*1a642130\n\t", "DUALANTENNAHEADINGA,USB3,0,48.0,FINESTEERING,2107,282313.600,02000000,d426,15824;INSUFFICIENT_OBS,NONE,0.000000000,0.000000000,0.000000000,0.0,0.000000000,0.000000000,\"\",0,0,0,0,00,00,00,00*80ae0999\n\t", "DUALANTENNAHEADINGA,USB3,0,48.0,FINESTEERING,2107,282314.100,02000000,d426,15824;SOL_COMPUTED,NARROW_FLOAT,-1.000000000,134.357482910,-58.416107178,0.0,360.000000000,180.000000000,\"631T\",15,6,6,5,04,00,20,03*a0098d17\n\t", "INSPVAXA,USB3,0,53.0,FINESTEERING,2107,282314.600,02000000,471d,15824;INS_ALIGNMENT_COMPLETE,INS_RTKFIXED,37.37064155403,126.72424590503,10.5186,22.3000,-0.2085,0.2358,0.0044,0.281854568,1.880117721,121.982291751,0.5806,0.3850,0.7206,0.1397,0.1125,0.0814,0.1439,0.1495,4.9286,0f000001,0*a4c93626\n\t", "DUALANTENNAHEADINGA,USB3,0,51.5,FINESTEERING,2107,282315.100,02000000,d426,15824;INSUFFICIENT_OBS,NONE,0.000000000,0.000000000,0.000000000,0.0,0.000000000,0.000000000,\"\",0,0,0,0,00,00,00,00*fb6d87b7\n\t", "DUALANTENNAHEADINGA,USB3,0,51.5,FINESTEERING,2107,282315.600,02000000,d426,15824;INSUFFICIENT_OBS,NONE,0.000000000,0.000000000,0.000000000,0.0,0.000000000,0.000000000,\"\",0,0,0,0,00,00,00,00*5226e786\n\t", "DUALANTENNAHEADINGA,USB3,0,48.0,FINESTEERING,2107,282316.100,02000000,d426,15824;SOL_COMPUTED,NARROW_FLOAT,-1.000000000,136.040298462,-67.713562012,0.0,360.000000000,180.000000000,\"631T\",17,7,7,5,04,00,20,03*78f64e13\n\t", "DUALANTENNAHEADINGA,USB3,0,48.0,FINESTEERING,2107,282316.600,02000000,d426,15824;SOL_COMPUTED,NARROW_FLOAT,-1.000000000,134.914855957,-67.706207275,0.0,360.000000000,180.000000000,\"631T\",16,7,7,5,04,00,20,03*7ca473fa\n\t", "DUALANTENNAHEADINGA,USB3,0,48.0,FINESTEERING,2107,282317.100,02000000,d426,15824;SOL_COMPUTED,L1_FLOAT,-1.000000000,88.879760742,-51.174438477,0.0,360.000000000,180.000000000,\"631T\",15,6,6,3,04,00,20,01*bfb98121\n\t", "DUALANTENNAHEADINGA,USB3,0,50.0,FINESTEERING,2107,282317.600,02000000,d426,15824;SOL_COMPUTED,L1_FLOAT,-1.000000000,88.347457886,-50.822692871,0.0,360.000000000,180.000000000,\"631T\",15,6,6,3,04,00,20,01*5e456794\n\t", "DUALANTENNAHEADINGA,USB3,0,50.0,FINESTEERING,2107,282318.100,02000000,d426,15824;INSUFFICIENT_OBS,NONE,0.000000000,0.000000000,0.000000000,0.0,0.000000000,0.000000000,\"\",0,0,0,0,00,00,00,00*a99f8f24\n\t", "DUALANTENNAHEADINGA,USB3,0,51.5,FINESTEERING,2107,282318.600,02000000,d426,15824;INSUFFICIENT_OBS,NONE,0.000000000,0.000000000,0.000000000,0.0,0.000000000,0.000000000,\"\",0,0,0,0,00,00,00,00*4bce61fe\n\t", "DUALANTENNAHEADINGA,USB3,0,51.5,FINESTEERING,2107,282319.100,02000000,d426,15824;SOL_COMPUTED,NARROW_FLOAT,-1.000000000,152.278427124,-75.170898438,0.0,360.000000000,65.870956421,\"631T\",16,7,7,5,04,00,20,03*bcd3d891\n\t", "DUALANTENNAHEADINGA,USB3,0,52.5,FINESTEERING,2107,282319.600,02000000,d426,15824;SOL_COMPUTED,NARROW_FLOAT,-1.000000000,152.142578125,-75.197906494,0.0,360.000000000,65.816017151,\"631T\",16,7,7,5,04,00,20,03*ee26bdb3\n\t", "DUALANTENNAHEADINGA,USB3,0,46.0,FINESTEERING,2107,282320.100,02000000,d426,15824;SOL_COMPUTED,NARROW_FLOAT,-1.000000000,137.905578613,-56.183776855,0.0,360.000000000,180.000000000,\"631T\",15,6,6,5,04,00,20,03*ad4a7336\n\t", "DUALANTENNAHEADINGA,USB3,0,46.0,FINESTEERING,2107,282320.600,02000000,d426,15824;SOL_COMPUTED,NARROW_FLOAT,-1.000000000,138.732131958,-57.118835449,0.0,360.000000000,180.000000000,\"631T\",15,6,6,5,04,00,20,03*b657a1f8\n\t", "DUALANTENNAHEADINGA,USB3,0,46.0,FINESTEERING,2107,282321.100,02000000,d426,15824;SOL_COMPUTED,NARROW_FLOAT,-1.000000000,138.171997070,-47.447601318,0.0,360.000000000,180.000000000,\"631T\",17,6,6,5,04,00,20,03*1bd00597\n\t", "DUALANTENNAHEADINGA,USB3,0,50.0,FINESTEERING,2107,282321.600,02000000,d426,15824;SOL_COMPUTED,NARROW_FLOAT,-1.000000000,138.598281860,-47.134765625,0.0,360.000000000,180.000000000,\"631T\",17,6,6,5,04,00,20,03*7418056f\n\t", "DUALANTENNAHEADINGA,USB3,0,50.0,FINESTEERING,2107,282322.100,02000000,d426,15824;SOL_COMPUTED,NARROW_FLOAT,-1.000000000,138.887161255,-70.719177246,0.0,360.000000000,133.361663818,\"631T\",17,7,7,5,04,00,20,03*5d30d365\n\t", "DUALANTENNAHEADINGA,USB3,0,50.5,FINESTEERING,2107,282322.600,02000000,d426,15824;SOL_COMPUTED,NARROW_FLOAT,-1.000000000,137.188095093,-70.605590820,0.0,360.000000000,140.173141479,\"631T\",17,7,7,5,04,00,20,02*f8e674e7\n\t", "DUALANTENNAHEADINGA,USB3,0,50.5,FINESTEERING,2107,282323.100,02000000,d426,15824;INSUFFICIENT_OBS,NONE,0.000000000,0.000000000,0.000000000,0.0,0.000000000,0.000000000,\"\",0,0,0,0,00,00,00,00*ed7be7e8\n\t", "DUALANTENNAHEADINGA,USB3,0,51.0,FINESTEERING,2107,282323.600,02000000,d426,15824;INSUFFICIENT_OBS,NONE,0.000000000,0.000000000,0.000000000,0.0,0.000000000,0.000000000,\"\",0,0,0,0,00,00,00,00*0f2a0932\n\t", "DUALANTENNAHEADINGA,USB3,0,51.0,FINESTEERING,2107,282324.100,02000000,d426,15824;INSUFFICIENT_OBS,NONE,0.000000000,0.000000000,0.000000000,0.0,0.000000000,0.000000000,\"\",0,0,0,0,00,00,00,00*2d8ea6a2\n\t", "DUALANTENNAHEADINGA,USB3,0,51.5,FINESTEERING,2107,282324.600,02000000,d426,15824;INSUFFICIENT_OBS,NONE,0.000000000,0.000000000,0.000000000,0.0,0.000000000,0.000000000,\"\",0,0,0,0,00,00,00,00*6f36fe3b\n\t", "DUALANTENNAHEADINGA,USB3,0,51.5,FINESTEERING,2107,282325.100,02000000,d426,15824;SOL_COMPUTED,NARROW_FLOAT,-1.000000000,140.911849976,-56.769714355,0.0,360.000000000,180.000000000,\"631T\",16,6,6,5,04,00,20,03*7a8a24a8\n\t", "DUALANTENNAHEADINGA,USB3,0,52.0,FINESTEERING,2107,282325.600,02000000,d426,15824;SOL_COMPUTED,NARROW_FLOAT,-1.000000000,140.545684814,-57.778442383,0.0,360.000000000,180.000000000,\"631T\",15,6,6,5,04,00,20,03*6799af52\n\t", "DUALANTENNAHEADINGA,USB3,0,51.5,FINESTEERING,2107,282326.100,02000000,d426,15824;INSUFFICIENT_OBS,NONE,0.000000000,0.000000000,0.000000000,0.0,0.000000000,0.000000000,\"\",0,0,0,0,00,00,00,00*e9297667\n\t", "DUALANTENNAHEADINGA,USB3,0,51.5,FINESTEERING,2107,282326.600,02000000,d426,15824;INSUFFICIENT_OBS,NONE,0.000000000,0.000000000,0.000000000,0.0,0.000000000,0.000000000,\"\",0,0,0,0,00,00,00,00*40621656\n\t", "DUALANTENNAHEADINGA,USB3,0,50.5,FINESTEERING,2107,282327.100,02000000,d426,15824;SOL_COMPUTED,NARROW_FLOAT,-1.000000000,125.369018555,-45.270568848,0.0,360.000000000,180.000000000,\"631T\",15,6,6,5,04,00,20,03*24996260\n\t", "DUALANTENNAHEADINGA,USB3,0,50.5,FINESTEERING,2107,282327.600,02000000,d426,15824;SOL_COMPUTED,NARROW_FLOAT,-1.000000000,125.215858459,-46.956237793,0.0,360.000000000,180.000000000,\"631T\",16,6,6,5,04,00,20,03*d17be84f\n\t", "DUALANTENNAHEADINGA,USB3,0,50.5,FINESTEERING,2107,282328.100,02000000,d426,15824;INSUFFICIENT_OBS,NONE,0.000000000,0.000000000,0.000000000,0.0,0.000000000,0.000000000,\"\",0,0,0,0,00,00,00,00*856e5927\n\t", "DUALANTENNAHEADINGA,USB3,0,51.5,FINESTEERING,2107,282328.600,02000000,d426,15824;INSUFFICIENT_OBS,NONE,0.000000000,0.000000000,0.000000000,0.0,0.000000000,0.000000000,\"\",0,0,0,0,00,00,00,00*8ccc8f55\n\t", "DUALANTENNAHEADINGA,USB3,0,51.5,FINESTEERING,2107,282329.100,02000000,d426,15824;SOL_COMPUTED,L1_FLOAT,-1.000000000,81.258789063,-50.005187988,0.0,360.000000000,180.000000000,\"631T\",16,6,6,3,04,00,20,01*7dc2aa1f\n\t", "DUALANTENNAHEADINGA,USB3,0,52.0,FINESTEERING,2107,282329.600,02000000,d426,15824;SOL_COMPUTED,L1_FLOAT,-1.000000000,80.095443726,-49.685882568,0.0,360.000000000,180.000000000,\"631T\",16,6,6,4,04,00,20,03*d7163941\n\t", "DUALANTENNAHEADINGA,USB3,0,52.0,FINESTEERING,2107,282331.100,02000000,d426,15824;INSUFFICIENT_OBS,NONE,0.000000000,0.000000000,0.000000000,0.0,0.000000000,0.000000000,\"\",0,0,0,0,00,00,00,00*4750fa4c\n\t", "DUALANTENNAHEADINGA,USB3,0,51.5,FINESTEERING,2107,282332.100,02000000,d426,15824;INSUFFICIENT_OBS,NONE,0.000000000,0.000000000,0.000000000,0.0,0.000000000,0.000000000,\"\",0,0,0,0,00,00,00,00*43ae011b\n\t", "DUALANTENNAHEADINGA,USB3,0,51.5,FINESTEERING,2107,282333.100,02000000,d426,15824;INSUFFICIENT_OBS,NONE,0.000000000,0.000000000,0.000000000,0.0,0.000000000,0.000000000,\"\",0,0,0,0,00,00,00,00*b9bcf60d\n\t", "DUALANTENNAHEADINGA,USB3,0,53.0,FINESTEERING,2107,282333.600,02000000,d426,15824;INSUFFICIENT_OBS,NONE,0.000000000,0.000000000,0.000000000,0.0,0.000000000,0.000000000,\"\",0,0,0,0,00,00,00,00*61a6c453\n\t", "DUALANTENNAHEADINGA,USB3,0,50.5,FINESTEERING,2107,282334.600,02000000,d426,15824;INSUFFICIENT_OBS,NONE,0.000000000,0.000000000,0.000000000,0.0,0.000000000,0.000000000,\"\",0,0,0,0,00,00,00,00*3bf1efde\n\t", "DUALANTENNAHEADINGA,USB3,0,53.0,FINESTEERING,2107,282335.600,02000000,d426,15824;SOL_COMPUTED,NARROW_FLOAT,-1.000000000,106.698776245,-65.583465576,0.0,360.000000000,180.000000000,\"631T\",15,7,7,5,04,00,20,03*5d10cc48\n\t", "DUALANTENNAHEADINGA,USB3,0,52.0,FINESTEERING,2107,282336.100,02000000,d426,15824;SOL_COMPUTED,L1_FLOAT,-1.000000000,75.314010620,-41.766326904,0.0,360.000000000,180.000000000,\"631T\",16,6,6,3,04,00,20,01*05518b35\n\t", "DUALANTENNAHEADINGA,USB3,0,52.0,FINESTEERING,2107,282336.600,02000000,d426,15824;SOL_COMPUTED,L1_FLOAT,-1.000000000,75.472106934,-40.715057373,0.0,360.000000000,180.000000000,\"631T\",16,6,6,3,04,00,20,01*06f451b5\n\t", "INSPVAXA,USB3,0,49.0,FINESTEERING,2107,282337.150,02000000,471d,15824;INS_ALIGNMENT_COMPLETE,INS_RTKFIXED,37.37060784122,126.72430452808,
